vi "Create Arbitrary Sequence [SEQ] Core.vi"(8 "error in (no error)":errorcluster, 9 "waveform handles array (empty)":i32[](array[numeric]), 10 "loop counts array (empty)":i32[](array[numeric]), 11 "CS++Fgen in":refnum<class "CS++Fgen.lvclass">) -> (0 "error out":errorcluster, 2 "sequence handle":i32, 3 "CS++Fgen out":refnum<class "CS++Fgen.lvclass">)   [LabVIEW 2013, in "CS++Fgen.lvlib" / "CS++Fgen.lvclass"]
doc: "An arbitrary sequence consists of multiple waveforms. For each waveform, you specify the number of times the function generator produces the waveform before proceeding to the next waveform. The number of times to repeat a specific waveform is called the loop count.\n \nThis VI creates an arbitrary sequence from an array of waveform handles and an array of corresponding loop counts. The VI returns a handle that identifies the sequence. You pass this handle to the IviFgen Configure Arbitrary Sequence [SEQ] VI to specify what arbitrary sequence you want the function generator to produce.\n\nNotes:\n\n(1) This VI is part of the IviFgenArbSeq [SEQ] extension group."
uses:
  CS++Fgen.lvclass
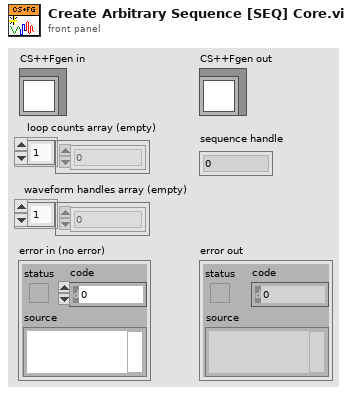
[diagram p1: front panel]
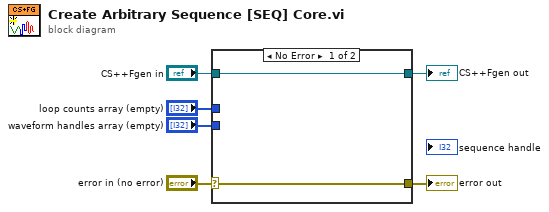
[diagram p0: block diagram]
diagram:
  n1 = case shown="No Error" "error in (no error)" {
    selector: "error in (no error)" -> [w7 w10]
    tunnel: [w7 w10] -> w5
    tunnel: [w8 w9] -> w3
    tunnel: "CS++Fgen in" -> [w8 w9]
    tunnel: "loop counts array (empty)" -> [_ _]
    tunnel: "waveform handles array (empty)" -> [_ _]
    frame No Error {
    }
    frame Error {
    }
  }
  "error out" <- w5
  "CS++Fgen out" <- w3
